vi "phase_timer_out.vi"(6 "FPGA I/O":refnum<k21>="LED0", 7 "Reset":bool, 8 "Channel number":u8, 9 "Output enable":bool[](array[boolean])=[FALSE, FALSE, FALSE, FALSE, FALSE, FALSE], 10 "Phase advance":T1[](array[typedef])=[0.0, 0.0, 0.0, 0.0, 0.0, 0.0], 11 "Initial phase":T1[](array[typedef])=[0.0, 0.0, 0.0, 0.0, 0.0, 0.0]) -> (2 "Pos edge":bool)   [LabVIEW 2014]
uses:
  Common/fractional_phase.ctl
  <vilib>/rvi/eio/common/nirviEmuTemplateMethod_errors.vi
  <vilib>/eio/EIONode/EIONode.xnode
panel:
  # "These phase arguments and the internal phase accumulator are represented as 1.32 fixed point (range 0 to one lsb short of 2.)  The output is one when the phase is less than one, and zero when the phase is greater.  That is, the phase in radians is pi times this number.  The phase advance defines the frequency to be (advance/2)*timebase.  The frequency resolution isn't quite as much as you might suppose with 32 bits, since the phase advance has 10 or more leading zeros."
  # "Used to index periods and output enable"
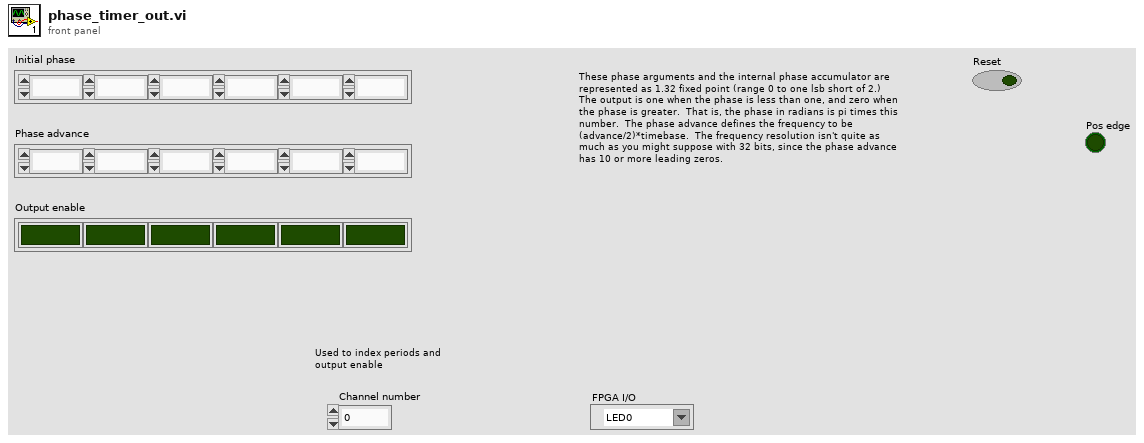
[diagram p1: front panel]
types:
  T1 = typedef "fractional_phase.ctl" = fxp<+,32,1>
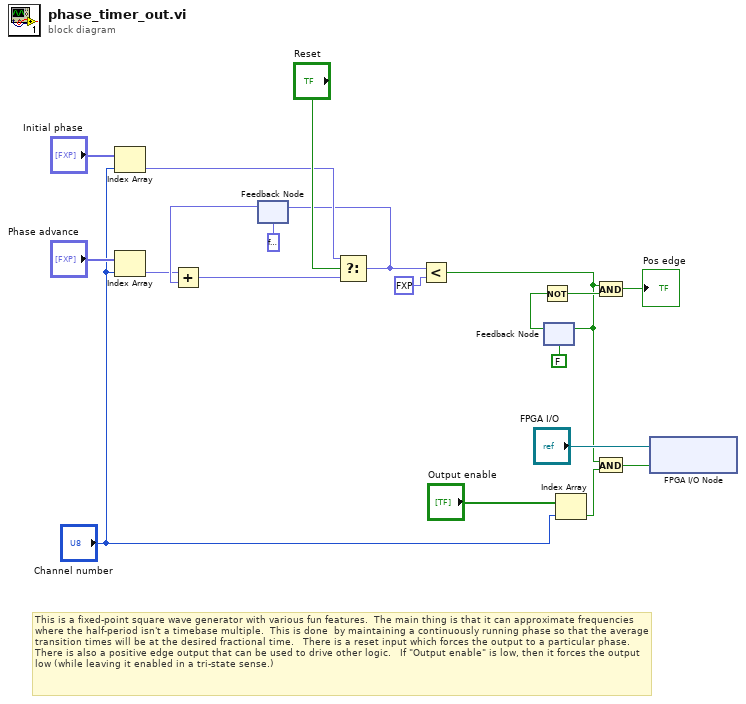
[diagram p0: block diagram]
diagram:
  # "This is a fixed-point square wave generator with various fun features.  The main thing is that it can approximate frequencies where the half-period isn't a timebase multiple.  This is done  by maintaining a continuously running phase so that the average transition times will be at the desired fractional time.   There is a reset input which forces the output to a particular phase.  There is also a positive edge output that can be used to drive other logic.   If \"Output enable\" is low, then it forces the output low (while leaving it enabled in a tri-state sense.)"
  n1 = Index Array(array="Initial phase", index="Channel number") -> (element=w6:T1)
  n2 = Index Array(array="Phase advance", index="Channel number") -> (element=w11:T1)
  n3 = feedback #1(T1 0.0 ("s? t:f")) -> (w16:fxp<+,48,1>)
  n4 = Add(x=w11, y=w16) -> (x+y=w5:fxp<+,48,1>)
  n5 = Select(t=w6, s="Reset", f=w5) -> (s? t:f=w3:fxp<+,48,1>)
  n6 = feedback-in #1(w3) -> ()
  n7 = Less?(x=w3, y=fxp<+,48,1> 1.0 ("element")) -> (x < y?=w2:bool)
  n8 = feedback #2(FALSE) -> (w20:bool)
  n9 = Not(x=w20) -> (.not. x?=w10:bool)
  n10 = feedback-in #2(w2) -> ()
  n11 = Index Array(array="Output enable", index="Channel number") -> (element=w18:bool)
  n12 = And(x=w2, y=w10) -> (x .and. y?=→"Pos edge":bool)
  n13 = And(x=w2, y=w18) -> (x .and. y?=w12:bool)
  n14 = xnode "FPGA I/O Node"("I/O Item"=w12, "FPGA I/O In"="FPGA I/O") -> ()  [unwired: 1 out]
